vi "Test_ReadFull.vi"() -> ()   [LabVIEW 2017, in "WordManipulationTests.lvlib"]
uses:
  WordManipulationTests.lvlib
  Utilities/Results_Trajectory.ctl
  Utilities/Results_MotionIO.ctl
  Utilities/Results_Faults.ctl
  SoftmotionClass/SoftmotionAxis/SoftmotionAxis.lvclass
  <vilib>/Motion/PropertyNodes/nimc.createStraightLineMoveInstance.axis.vi
  <vilib>/Motion/PropertyNodes/nimc.destroyInterfaceInstance.vi
  <resource>/objmgr/nimcai.rc
  Utilities/WordManipulationLibrary.lvlib
panel:
  out "Fault Data":T1[](array[typedef])
  out "Motion I/O":T2[](array[typedef])
  out "Feedback":T3[](array[typedef])
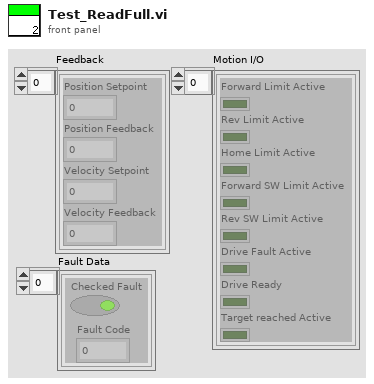
[diagram p1: front panel]
types:
  T1 = typedef "WordManipulationLibrary.lvlib/Results_Faults.ctl" = cluster{"Checked Fault":bool, "Fault Code":i32}
  T2 = typedef "WordManipulationLibrary.lvlib/Results_MotionIO.ctl" = cluster{"Forward Limit Active":bool, "Rev Limit Active":bool, "Home Limit Active":bool, "Forward SW Limit Active":bool, "Rev SW Limit Active":bool, "Drive Fault Active":bool, "Drive Ready":bool, "Target reached Active":bool}
  T3 = typedef "WordManipulationLibrary.lvlib/Results_Trajectory.ctl" = cluster{"Position Setpoint":dbl, "Position Feedback":dbl, "Velocity Setpoint":dbl, "Velocity Feedback":dbl}
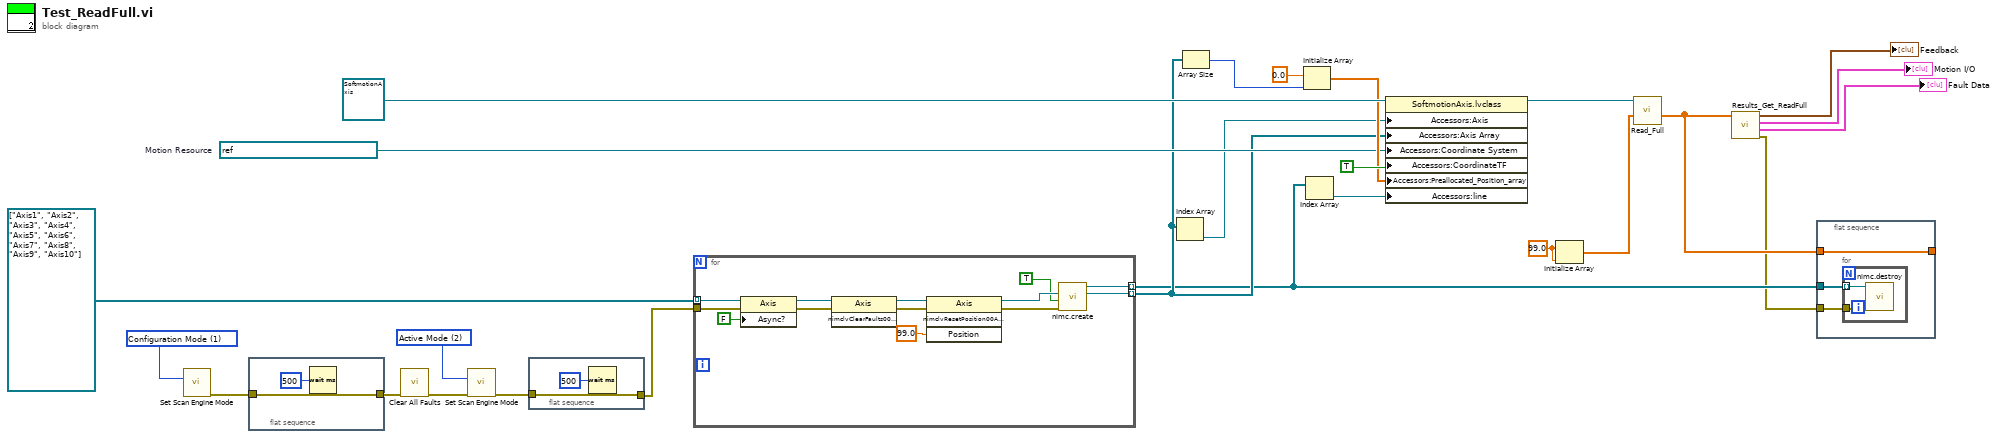
[diagram p0: block diagram]
diagram:
  w8 = 99.0 ("element")
  w14 = 2 items=["Configuration Mode"=1, "Active Mode"=2] ("mode (Active Mode)")
  w16 = 1 items=["Configuration Mode"=1, "Active Mode"=2] ("mode (Active Mode)")
  w22 = refnum<k21> "nism://My Computer/Cord1"  # Motion Resource
  n1 = call <vilib>:"Set Scan Engine Mode.vi"("mode (Active Mode)"=w16) -> ("error out"=w13:errorcluster)  [unwired: 14 in]
  n2 = flat-sequence {
    tunnel: [w27] -> w12
    tunnel: w13 -> [w27]
    frame #0 {
      n3 = Wait (ms)(milliseconds to wait=u32 500) -> ()  [unwired: 1 out]
    }
  }
  n4 = call <vilib>:"Clear All Faults.vi"("error in (no error)"=w12) -> ("error out"=w11:errorcluster)  [unwired: 10 in]
  n5 = call <vilib>:"Set Scan Engine Mode.vi"("mode (Active Mode)"=w14, "error in (no error)"=w11) -> ("error out"=w10:errorcluster)  [unwired: 13 in]
  n6 = flat-sequence {
    tunnel: [w29] -> w15
    tunnel: w10 -> [w29]
    frame #0 {
      n7 = Wait (ms)(milliseconds to wait=u32 500) -> ()  [unwired: 1 out]
    }
  }
  n8 = for {
    tunnel: refnum<k21>[] ["Axis1", "Axis2", "Axis3", "Axis4", "Axis5", "Axis6", "Axis7", "Axis8", "Axis9", "Axis10"] ("Axis Array") -> [w42] mode=indexing
    tunnel: [w38] -> w17 mode=indexing
    tunnel: [w37] -> w5 mode=indexing
    tunnel: w15 -> [w36]
    n9 = property class="Axis"(reference=w42, error in=w36, "Async?"=FALSE) -> (reference out=w35:refnum<k21>, error out=w33:errorcluster)
    n10 = invoke class="Axis" method="nimclvClearFaults00A10001"(reference=w35, error in=w33) -> (reference out=w34:refnum<k21>, error out=w32:errorcluster)  [unwired: 1 in, 1 out]
    n11 = invoke class="Axis" method="nimclvResetPosition00A10001"(reference=w34, error in=w32, "Position"=99.0) -> (reference out=w40:refnum<k21>, error out=w31:errorcluster)  [unwired: 1 in, 2 out]
    n12 = call-poly <vilib>:"nimc.create.vi"("error in"=w31, "async?"=TRUE, "axis"=w40) -> ("axis out"=w38:refnum<k21>, "line"=w37:refnum<k20>)  [unwired: 6 in, 1 out]
  }
  n13 = Index Array(array=w17) -> (element=w18:refnum<k21>)  [unwired: 1 in]
  n14 = Array Size(array=w17) -> (size(s)=w21:i32)
  n15 = Initialize Array(0.0 ("element"), w21) -> (w23:dbl[])
  n16 = Index Array(array=w5) -> (element=w19:refnum<k20>)  [unwired: 1 in]
  n17 = property class="SoftmotionAxis.lvclass"(reference=refnum<class "SoftmotionAxis.lvclass"> refnum ("SoftmotionAxis in"), "Accessors:Axis"=w18, "Accessors:Axis Array"=w17, "Accessors:Coordinate System"=w22, "Accessors:CoordinateTF"=TRUE ("CoordinateTF"), "Accessors:Preallocated_Position_array"=w23, "Accessors:line"=w19) -> (reference out=w9:refnum<class "SoftmotionAxis.lvclass">)  [unwired: 1 in, 1 out]
  n18 = Initialize Array(w8, w8) -> (w7:dbl[])
  n19 = call-dynamic "Read_Full.vi"("Results Array In"=w7, "SoftmotionAxis in"=w9) -> ("appended array"=w6:dbl[])  [unwired: 7 in, 2 out]
  n20 = call "Results_Get_ReadFull.vi"("appended array"=w6) -> ("error out"=w4:errorcluster, "Fault Data"=→"Fault Data":T1[], "Motion I/O"=→"Motion I/O":T2[], "Feedback"=→"Feedback":T3[])  [unwired: 7 in]
  n21 = flat-sequence {
    tunnel: w5 -> [w46]
    tunnel: [w45] -> _
    tunnel: w6 -> [w45]
    tunnel: w4 -> [w44]
    frame #0 {
      n22 = for {
        tunnel: w46 -> [w48] mode=indexing
        tunnel: w44 -> [w47]
        n23 = call-poly <vilib>:"nimc.destroy.vi"("error in"=w47, "motion handle"=w48) -> ()  [unwired: 9 in, 1 out]
      }
    }
  }
